vi "G-CLI-Build.vi"() -> ()   [LabVIEW 2017]
uses:
  <vilib>/addons/_JKI Toolkits/Caraya/run-tests/Run Test (Scalar Path).vi
  <vilib>/Wiresmith Technology/G CLI/CLI Class/CLI.lvclass
  <vilib>/JKI/VIPM API/VIPM API_vipm_api.lvlib
  <vilib>/addons/_JKI Toolkits/Caraya/Caraya.lvlib
panel:
  in  "Build Regardless of G-CLI Error":bool
  out "build error":errorcluster
  out "g-cli error":errorcluster
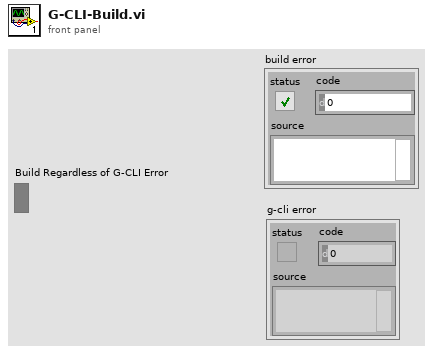
[diagram p1: front panel]
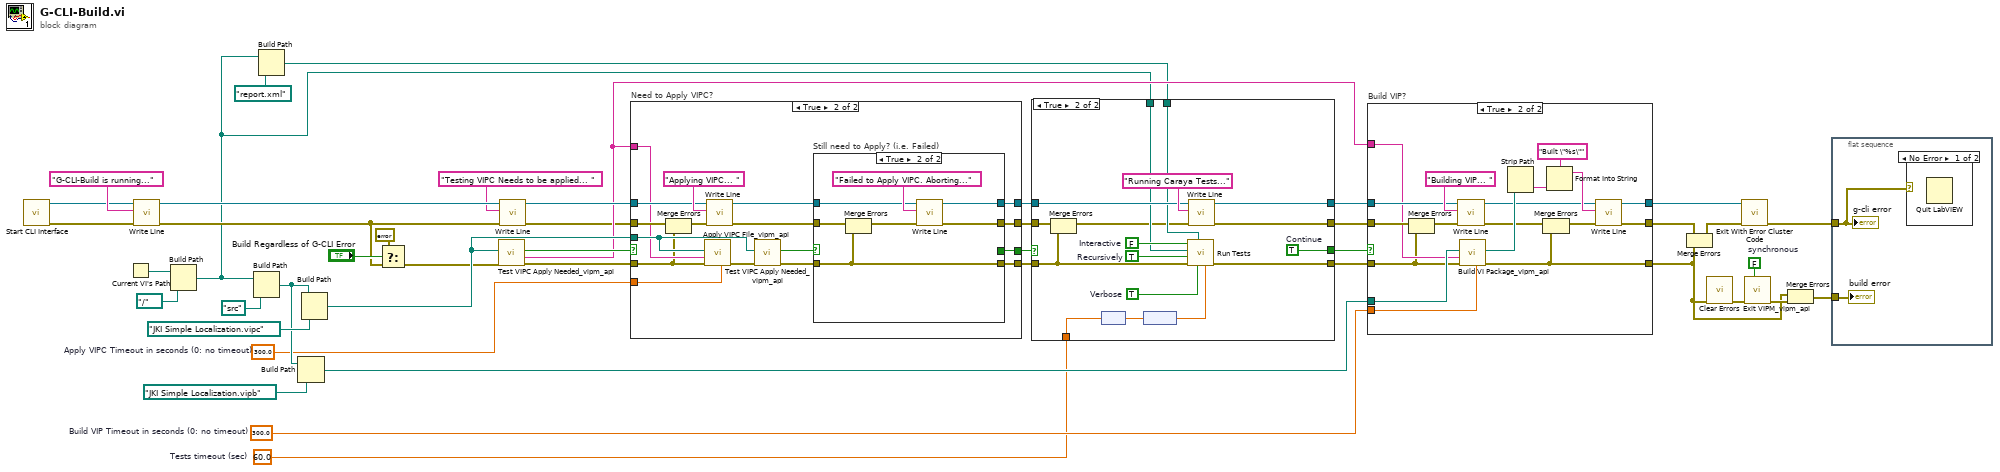
[diagram p0: block diagram]
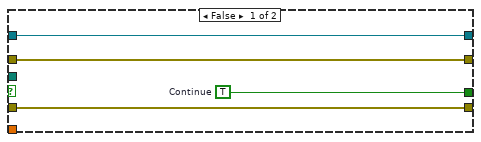
[diagram p5: hidden frame]
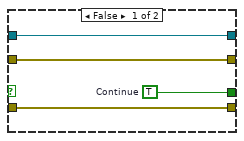
[diagram p6: hidden frame]
diagram:
  w5 = 60.0  # Tests timeout (sec)
  w18 = FALSE  # synchronous
  w23 = 300.0  # Build VIP Timeout in seconds (0: no timeout)
  w32 = 300.0  # Apply VIPC Timeout in seconds (0: no timeout)
  n1 = call <vilib>:"Start CLI Interface.vi"() -> ("error out"=w45:errorcluster, "CLI out"=w43:refnum<class "CLI.lvclass">)  [unwired: 8 in, 2 out]
  n2 = Current VI's Path() -> (path=w30:path)
  n3 = call <vilib>:"Write Line.vi"("error in (no error)"=w45, "Text to Write"="G-CLI-Build is running...", "CLI in"=w43) -> ("error out"=w14:errorcluster, "CLI out"=w42:refnum<class "CLI.lvclass">)  [unwired: 7 in]
  n4 = Build Path(base path=w30, name or relative path=path "../.." ("base path")) -> (appended path=w6:path)
  n5 = Build Path(base path=w6, name or relative path=path "src" ("base path")) -> (appended path=w33:path)
  n6 = Build Path(base path=w6, name or relative path=path "report.xml" ("base path")) -> (appended path=w7:path)
  n7 = Build Path(base path=w33, name or relative path=path "JKI Simple Localization.vipb" ("base path")) -> (appended path=w24:path)
  n8 = Build Path(base path=w33, name or relative path=path "JKI Simple Localization.vipc" ("base path")) -> (appended path=w35:path)
  n9 = Select(t=errorcluster {"status"=FALSE, "code"=0, "source"=""}, s="Build Regardless of G-CLI Error", f=w14) -> (s? t:f=w27:errorcluster)
  n10 = call <vilib>:"Test VIPC Apply Needed_vipm_api.vi"("error in (no error)"=w27, "VIPC File Path"=w35) -> ("error out"=w37:errorcluster, "VIPC File LabVIEW Version"=w20:string, "Need to Apply?"=w39:bool)  [unwired: 7 in]
  n11 = call <vilib>:"Write Line.vi"("error in (no error)"=w14, "Text to Write"="Testing VIPC Needs to be applied... ", "CLI in"=w42) -> ("error out"=w13:errorcluster, "CLI out"=w38:refnum<class "CLI.lvclass">)  [unwired: 7 in]
  n12 = case "Need to Apply VIPC?" shown="True" w39 {
    tunnel: w13 -> [w48 w65]
    tunnel: w38 -> [w49 w64]
    tunnel: w35 -> [_ w62]
    tunnel: w37 -> [w47 w50]
    tunnel: [w48 w56] -> w10
    tunnel: [w49 w58] -> w9
    tunnel: [w47 w53] -> w11
    tunnel: w32 -> [_ w61]
    tunnel: w20 -> [_ w60]
    tunnel: [w46 w54] -> w12
    frame False {
      w46 = TRUE  # Continue
    }
    frame True {
      n13 = Merge Errors(w65, w50) -> (w51:errorcluster)
      n14 = call <vilib>:"Apply VIPC File_vipm_api.vi"("Timeout in seconds (0: no timeout)"=w61, "error in (no error)"=w50, "LabVIEW Version"=w60, "VIPC File"=w62) -> ("error out"=w63:errorcluster)  [unwired: 7 in]
      n15 = call <vilib>:"Write Line.vi"("error in (no error)"=w51, "Text to Write"="Applying VIPC... ", "CLI in"=w64) -> ("error out"=w57:errorcluster, "CLI out"=w59:refnum<class "CLI.lvclass">)  [unwired: 7 in]
      n16 = call <vilib>:"Test VIPC Apply Needed_vipm_api.vi"("error in (no error)"=w63, "VIPC File Path"=w62) -> ("error out"=w52:errorcluster, "Need to Apply?"=w55:bool)  [unwired: 7 in, 1 out]
      n17 = case "Still need to Apply? (i.e. Failed)" shown="True" w55 {
        tunnel: w59 -> [w70 w76]
        tunnel: [w70 w75] -> w58
        tunnel: w57 -> [w69 w74]
        tunnel: [w69 w73] -> w56
        tunnel: [w68 _] -> w54
        tunnel: [w67 w71] -> w53
        tunnel: w52 -> [w67 w71]
        frame False {
          w68 = TRUE  # Continue
        }
        frame True {
          n18 = Merge Errors(w74, w71) -> (w72:errorcluster)
          n19 = call <vilib>:"Write Line.vi"("error in (no error)"=w72, "Text to Write"="Failed to Apply VIPC. Aborting...", "CLI in"=w76) -> ("error out"=w73:errorcluster, "CLI out"=w75:refnum<class "CLI.lvclass">)  [unwired: 7 in]
        }
      }
    }
  }
  n20 = case shown="True" w12 {
    tunnel: w11 -> [w78 w81]
    tunnel: w10 -> [w79 w95]
    tunnel: w9 -> [w80 w96]
    tunnel: w7 -> [_ w94]
    tunnel: w6 -> [_ w92]
    tunnel: w5 -> [_ w90]
    tunnel: [w78 w86] -> w4
    tunnel: [w80 w85] -> w2
    tunnel: [w79 w84] -> w3
    tunnel: [_ w83] -> w1
    frame False {
    }
    frame True {
      w83 = TRUE  # Continue
      w87 = TRUE  # Verbose
      w91 = TRUE  # Recursively
      w93 = FALSE  # Interactive
      n21 = Merge Errors(w95, w81) -> (w82:errorcluster)
      n22 = node(w90) -> (w89:dbl[unit])
      n23 = node(w89) -> (w88:dbl)
      n24 = call-poly <vilib>:"Run Tests.vi"("timeout (2000 ms)"=w88, "Verbose"=w87, "Report Path"=w94, "error in"=w81, "Inspect Recursively (T)"=w91, "Test Path"=w92, "Interactive (T)"=w93) -> ("error out"=w86:errorcluster)  [unwired: 4 in]
      n25 = call <vilib>:"Write Line.vi"("error in (no error)"=w82, "Text to Write"="Running Caraya Tests...", "CLI in"=w96) -> ("error out"=w84:errorcluster, "CLI out"=w85:refnum<class "CLI.lvclass">)  [unwired: 7 in]
    }
  }
  n26 = case "Build VIP?" shown="True" w1 {
    tunnel: w4 -> [w98 w103]
    tunnel: w2 -> [w100 w117]
    tunnel: w3 -> [w99 w116]
    tunnel: [w99 w106] -> w22
    tunnel: [w100 w108] -> w21
    tunnel: [w98 w101] -> w15
    tunnel: w24 -> [_ w115]
    tunnel: w23 -> [_ w114]
    tunnel: w20 -> [_ w105]
    frame False {
    }
    frame True {
      n27 = Merge Errors(w116, w103) -> (w104:errorcluster)
      n28 = call <vilib>:"Write Line.vi"("error in (no error)"=w104, "Text to Write"="Building VIP... ", "CLI in"=w117) -> ("error out"=w107:errorcluster, "CLI out"=w109:refnum<class "CLI.lvclass">)  [unwired: 7 in]
      n29 = call <vilib>:"Build VI Package_vipm_api.vi"("Timeout in seconds (0: no timeout)"=w114, "error in (no error)"=w103, "LabVIEW Version"=w105, "Path to VIPB File"=w115) -> ("error out"=w101:errorcluster, "Build Output"=w113:path)  [unwired: 6 in]
      n30 = Strip Path(path=w113) -> (name=w112:string)  [unwired: 1 out]
      n31 = Merge Errors(w107, w101) -> (w102:errorcluster)
      n32 = Format Into String(format string="Built \"%s\"" ("Text to Write"), w112) -> (resulting string=w110:string)  [unwired: 2 in, 1 out]
      n33 = call <vilib>:"Write Line.vi"("error in (no error)"=w102, "Text to Write"=w110, "CLI in"=w109) -> ("error out"=w106:errorcluster, "CLI out"=w108:refnum<class "CLI.lvclass">)  [unwired: 7 in]
    }
  }
  n34 = Merge Errors(w22, w15) -> (w29:errorcluster)
  n35 = call <vilib>:"Clear Errors.vi"("error in (no error)"=w15) -> ("error out"=w17:errorcluster)  [unwired: 5 in, 1 out]
  n36 = call <vilib>:"Exit With Error Cluster Code.vi"("error in (no error)"=w29, "CLI in"=w21) -> ("error out"=w25:errorcluster)  [unwired: 9 in]
  n37 = call <vilib>:"Exit VIPM_vipm_api.vi"("synchronous? (T)"=w18, "error in (no error)"=w17) -> ("error out"=w19:errorcluster)  [unwired: 9 in]
  n38 = Merge Errors(w15, w19) -> (w16:errorcluster)
  n39 = flat-sequence {
    tunnel: w25 -> [w119]
    tunnel: w16 -> [w120]
    frame #0 {
      n40 = case shown="No Error" w119 {
        frame No Error {
          n41 = Quit LabVIEW() -> ()  [unwired: 1 in]
        }
        frame Error {
        }
      }
      "g-cli error" <- w119
      "build error" <- w120
    }
  }
